vi "Bottom Shooter Interpolation.vi"(11 "Distance":dbl) -> (3 "interpolation value":dbl format="%0.2f")   [LabVIEW 2019]
uses:
  <vilib>/Analysis/NI_AALPro.lvlib
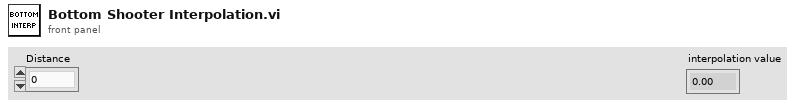
[diagram p1: front panel]
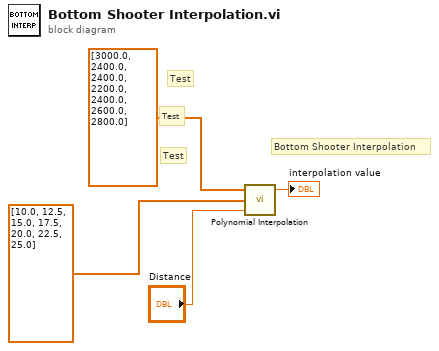
[diagram p0: block diagram]
diagram:
  # "Bottom Shooter Interpolation"
  # "Test"
  # "Test"
  # "Test"
  n1 = call <vilib>:"Polynomial Interpolation.vi"("x value"="Distance", "X"=dbl[] [10.0, 12.5, 15.0, 17.5, 20.0, 22.5, 25.0], "Y"=dbl[] [3000.0, 2400.0, 2400.0, 2200.0, 2400.0, 2600.0, 2800.0]) -> ("interpolation value"=→"interpolation value":dbl)  [unwired: 2 out]
